vi "Z6_Beamline.Calc Southtower State.vi"(0 "i ref in":refnum<vi>, 5 "error in (no error)":errorcluster) -> (14 "i ref out":refnum<vi>, 19 "error out":errorcluster)   [LabVIEW 2014, in "Z6_Beamline.lvlib"]
doc: "This VI calculates the Southtower state of the Z6 Beamline."
uses:
  Z6_Beamline.lvlib
  PH_StatusHandler/PH_StatusHandler.Status.ctl
  PH_Common/PH_Common.lvlib
  PH_StatusHandler/PH_StatusHandler.lvlib
  PH_BL-Master/PH_BL-Master.lvlib
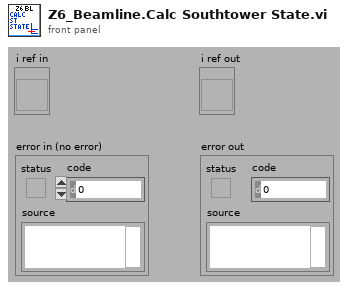
[diagram p1: front panel]
types:
  T1 = typedef "PH_StatusHandler.lvlib/PH_StatusHandler.Status.ctl" = i16
  T2 = typedef "Z6_Beamline.lvlib/Z6_Beamline.i attribute.ctl" = cluster{"Subs ok GUI Refs":T3, "Refs BL Northtower":refnum<vi>[], "Refs BL Southtower":refnum<vi>[], "Refs BL 100TW COS":refnum<vi>[], "State Subsystems":cluster{"Northtower":bool, "Southtower":bool, "Frontends":bool, "100TW COS":bool}, "Z6 Beamline Status Subscriber Information":T4, "Color State PHELIX":i16}
  T3 = typedef "Z6_Beamline.lvlib/Z6_Beamline.Subsystem ok GUI Refs.ctl" = cluster{"Northtower ok":refnum<vi>, "Southtower ok":refnum<vi>, "Frontends ok":refnum<vi>, "100TW COS ok":refnum<vi>}
  T4 = typedef "Z6_Beamline.lvlib/Z6_Beamline.Status Subscriber Information.ctl" = cluster{"BL Z6 Shutter":T5, "CH 10":T5, "CH 11":T5, "ST Flip Cam":T5, "ST Flip DB":T5, "BL Z6 Dump":T5}
  T5 = typedef "PH_BL-Master.lvlib/PH_BL-Master.Status Subscriber Information.ctl" = cluster{"Index of element":i32, "Attributeset":T6}
  T6 = typedef "PH_BL-Master.lvlib/PH_BL-Master.Attribute Set.ctl" = enum16{"Boolean Status Service Subscriber", "Picture Status Service Subscriber"}
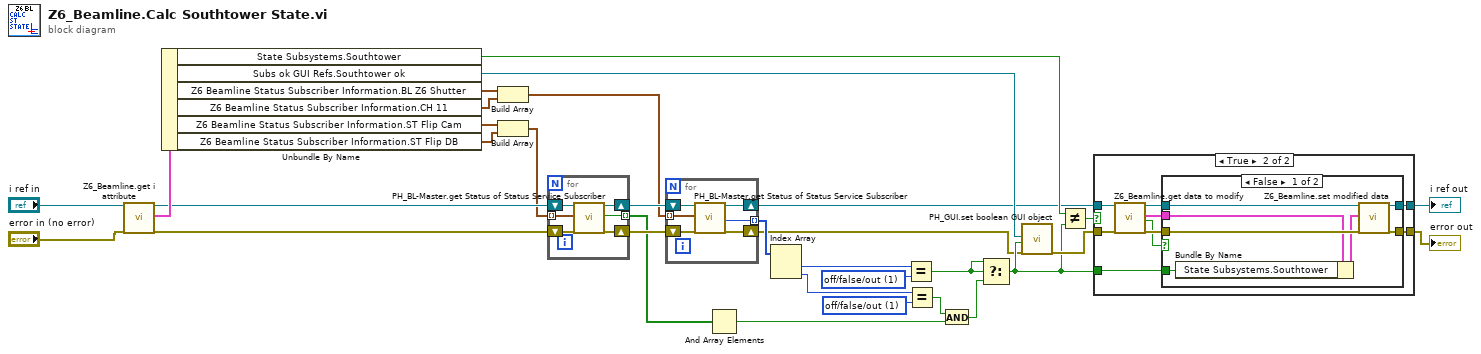
[diagram p0: block diagram]
diagram:
  w22 = T1 1 items=["no info", "off/false/out", "on/true/in", "Failure", "Alarm", "Status 1", "Status 2", "Status 3"] ("element")
  w23 = T1 1 items=["no info", "off/false/out", "on/true/in", "Failure", "Alarm", "Status 1", "Status 2", "Status 3"] ("element")
  n1 = call "Z6_Beamline.get i attribute.vi"("i ref in"="i ref in", "error in (no error)"="error in (no error)") -> ("i ref out"=w10:refnum<vi>, "i attribute"=w32:T2, "error out"=w11:errorcluster)  [unwired: 15 in]
  n2 = Unbundle By Name(w32) -> ("State Subsystems.Southtower"=w29:bool, "Subs ok GUI Refs.Southtower ok"=w31:refnum<vi>, "Z6 Beamline Status Subscriber Information.BL Z6 Shutter"=w7:T5, "Z6 Beamline Status Subscriber Information.CH 11"=w6:T5, "Z6 Beamline Status Subscriber Information.ST Flip Cam"=w4:T5, "Z6 Beamline Status Subscriber Information.ST Flip DB"=w3:T5)
  n3 = Build Array(w7, w6) -> (w5:T5[])
  n4 = Build Array(w4, w3) -> (w2:T5[])
  n5 = for {
    tunnel: [w33] -> w14 mode=indexing
    tunnel: w2 -> [w34] mode=indexing
    shift-right: [w37] -> w17
    shift-left: w11 -> [w36]
    shift-right: [w38] -> w18
    shift-left: w10 -> [w35]
    n6 = call "PH_BL-Master.get Status of Status Service Subscriber.vi"("i ref in"=w35, "Wanted Status Subscriber Information"=w34, "error in (no error)"=w36) -> ("i ref out"=w38:refnum<vi>, "on/true/in?"=w33:bool, "error out"=w37:errorcluster)  [unwired: 11 in, 3 out]
  }
  n7 = for {
    tunnel: w5 -> [w40] mode=indexing
    shift-right: [w43] -> w8
    shift-left: w17 -> [w44]
    shift-right: [w41] -> w9
    shift-left: w18 -> [w42]
    tunnel: [w39] -> w25 mode=indexing
    n8 = call "PH_BL-Master.get Status of Status Service Subscriber.vi"("i ref in"=w42, "Wanted Status Subscriber Information"=w40, "error in (no error)"=w44) -> ("i ref out"=w41:refnum<vi>, "Status"=w39:T1, "error out"=w43:errorcluster)  [unwired: 11 in, 3 out]
  }
  n9 = And Array Elements(Boolean array=w14) -> (logical AND=w1:bool)
  n10 = Index Array(array=w25) -> (element #1=w24:T1, element #2=w20:T1)  [unwired: 2 in]
  n11 = Equal?(x=w24, y=w23) -> (x = y?=w21:bool)
  n12 = Equal?(x=w20, y=w22) -> (x = y?=w16:bool)
  n13 = And(x=w16, y=w1) -> (x .and. y?=w15:bool)
  n14 = Select(t=w21, s=w21, f=w15) -> (s? t:f=w19:bool)
  n15 = call "PH_GUI.set boolean GUI object.vi"("Boolean Knob GUI Ref"=w31, "Value"=w19, "error in (no error)"=w8) -> ("error out"=w27:errorcluster)  [unwired: 16 in]
  n16 = Not Equal?(x=w29, y=w19) -> (x != y?=w30:bool)
  n17 = case shown="True" w30 {
    tunnel: w9 -> [w46 w51]
    tunnel: [w46 w50] -> w28
    tunnel: w27 -> [w45 w49]
    tunnel: [w45 w48] -> w26
    tunnel: w19 -> [_ w47]
    frame False {
    }
    frame True {
      n18 = call "Z6_Beamline.get data to modify.vi"("i ref in"=w51, "error in (no error)"=w49) -> ("i ref out"=w54:refnum<vi>, "i attribute"=w52:T2, "timed out"=w53:bool, "error out"=w55:errorcluster)  [unwired: 14 in]
      n19 = case shown="False" w53 {
        tunnel: w55 -> [w62 w63]
        tunnel: w54 -> [w61 w64]
        tunnel: [w60 w63] -> w48
        tunnel: [w59 w64] -> w50
        tunnel: w52 -> [w58 _]
        tunnel: w47 -> [w56 _]
        frame False {
          n20 = Bundle By Name(cluster=w58, "State Subsystems.Southtower"=w56) -> (w57:T2)
          n21 = call "Z6_Beamline.set modified data.vi"("i ref in"=w61, "i attribute"=w57, "error in (no error)"=w62) -> ("i ref out"=w59:refnum<vi>, "error out"=w60:errorcluster)  [unwired: 15 in]
        }
        frame True {
        }
      }
    }
  }
  "i ref out" <- w28
  "error out" <- w26
